vi "RT-TrapTest.vi"() -> ()   [LabVIEW 2010]
uses:
  <vilib>/userDefined/High Color/nirio_resource_hc.ctl
  <vilib>/rvi/interface/nirviOpenFPGA/nirviOpenFPGA.xnode
  C:/Users/HAGAR-IV/Desktop/HAGAR-V_Steuerung/Users/HAGAR-IV/Desktop/Johnny/pertrasgc fpga/FPGA-Trap-Test.vi
  <vilib>/rvi/ClientSDK/nirviWhatTheDeviceIsDoing.ctl
  <vilib>/rvi/interface/nirviReadWriteControl/nirviReadWriteControl.xnode
  <vilib>/rvi/interface/common/niFpgaNodeNameForErrorReporting.ctl
  <vilib>/rvi/errors/niLvFpgaWhatHappensToTopLevelVI.ctl
  <vilib>/rvi/interface/nirviMethod/nirviMethod.xnode
  <vilib>/rvi/interface/nirviCloseFPGA/nirviCloseFPGA.xnode
  <vilib>/FPGAPlugInAG/cRIO-9114/niLvFpga_Open_cRIO-9114.vi
  <vilib>/rvi/interface/common/dynamic/niFpgaDynamicAddResources.vi
  <vilib>/Utility/error.llb/Error Cluster From Error Code.vi
  <vilib>/rvi/errors/niLvFpgaAdjustHostInterfaceError.vi
  <vilib>/FPGAPlugInAG/Dynamic/niLvFpga_Close_Dynamic.vi
  NiFpgaLv.dll
panel:
  out "XY Graph":cluster{dbl[], dbl[]}(graph)
  out "Widrschtond":dbl
  in  "WerteMitteln":i32
  out "TempTrap":dbl
  in  "T(R)Koeff0":dbl=-251.0
  in  "T(R)Koeff2":dbl=-0.96
  in  "T(R)Koeff1":dbl=46.0
  out "WiderstandHeizdraht":dbl
  in  "Spannung":dbl=4.3
  in  "Präzisionswidrschtond":dbl=8.43
  in  "stop":bool
  in  "5VTrap1":bool
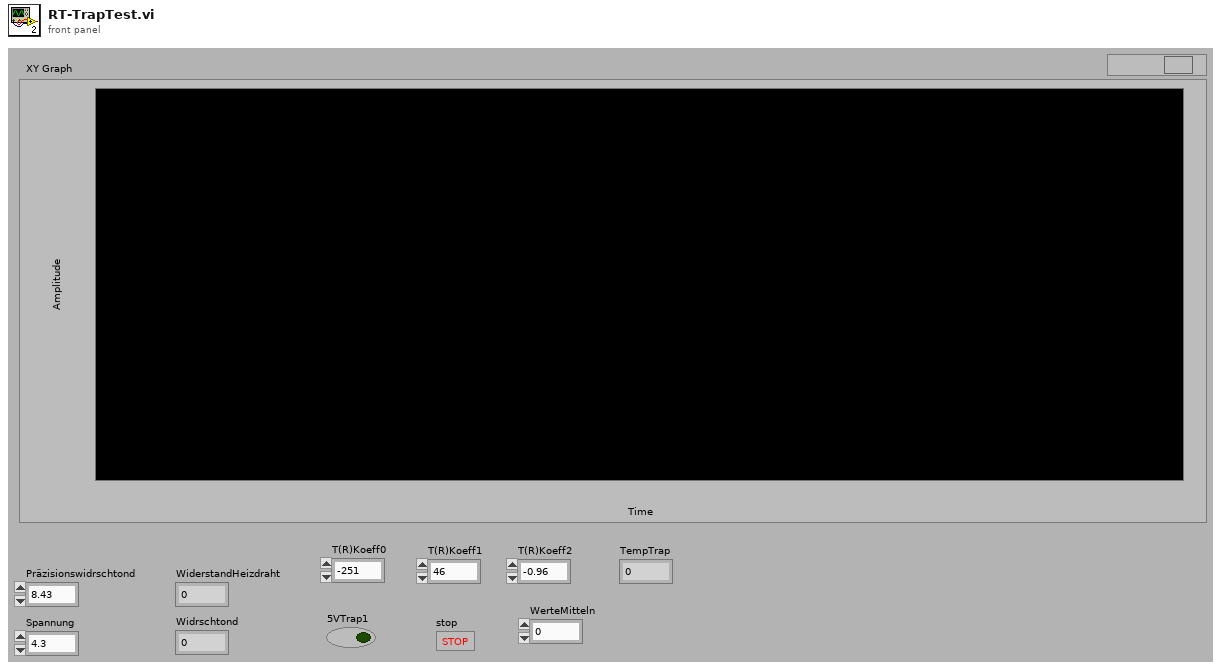
[diagram p1: front panel]
types:
  T1 = typedef "niFpgaNodeNameForErrorReporting.ctl" = enum16{"Open FPGA VI Reference", "Read/Write Control", "Invoke Method: Abort", "Invoke Method: Acknowledge IRQ", "Invoke Method: Download", "Invoke Method: FIFO.Configure", "Invoke Method: FIFO.Read", "Invoke Method: FIFO.Start", "Invoke Method: FIFO.Stop", "Invoke Method: FIFO.Write", "Invoke Method: Reset", "Invoke Method: Run", "Invoke Method: Wait on IRQ", "Close FPGA VI Reference"}
  T2 = typedef "niLvFpgaWhatHappensToTopLevelVI.ctl" = enum16{"top level VI scripted behind XNode", "top level VI inlined behind XNode"}
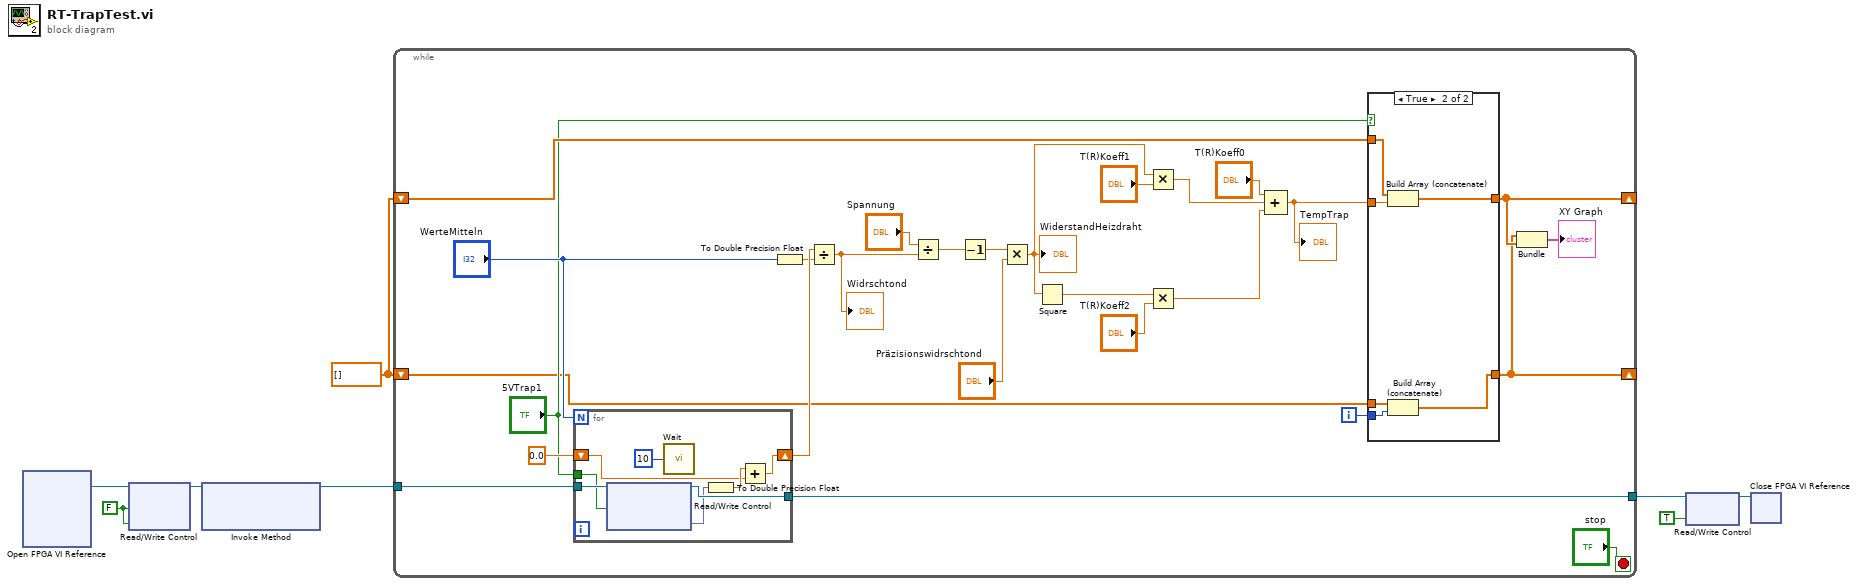
[diagram p0: block diagram]
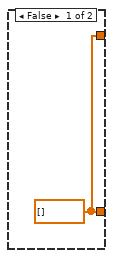
[diagram p2: hidden frame]
diagram:
  w1 = dbl[] []
  w7 = FALSE ("5VTrap1")
  n1 = xnode "Open FPGA VI Reference"() -> ("FPGA VI Reference Out"=w8:refnum<k20>)  [unwired: 2 in, 1 out]
  n2 = xnode "Read/Write Control"("FPGA VI Reference In"=w8, "5VTrap1"=w7, "stop"=w7) -> ("FPGA VI Reference Out"=w6:refnum<k20>)  [unwired: 1 in, 1 out]
  n3 = xnode "Invoke Method"("FPGA VI Reference In"=w6) -> ("FPGA VI Reference Out"=w5:refnum<k20>)  [unwired: 2 in, 1 out]
  n4 = while {
    tunnel: w5 -> [w35]
    tunnel: [w33] -> w4
    shift-right: [w13] -> _
    shift-left: w1 -> [w15]
    shift-right: [w9] -> _
    shift-left: w1 -> [w12]
    i -> [w11]
    stop <- "stop" stop-if-true
    n5 = for {
      N: "WerteMitteln" -> [_]
      tunnel: w35 -> [w50]
      tunnel: [w49] -> w33
      shift-right: [w45] -> w19
      shift-left: 0.0 -> [w46]
      tunnel: "5VTrap1" -> [w43]
      n6 = xnode "Read/Write Control"("FPGA VI Reference In"=w50, "5VTrap1"=w43) -> ("FPGA VI Reference Out"=w49:refnum<k20>, "AIWidrTrap1"=w48:fxp<+/-,26,5>)  [unwired: 1 in, 1 out]
      n7 = call "Wait"("Count(mSec)"=u32 10) -> ()  [unwired: 1 out]
      n8 = To Double Precision Float(number=w48) -> (double precision float=w47:dbl)
      n9 = Add(x=w47, y=w46) -> (x+y=w45:dbl)
    }
    n10 = To Double Precision Float(number="WerteMitteln") -> (double precision float=w18:dbl)
    n11 = Divide(x=w19, y=w18) -> (x/y=w17:dbl)
    "Widrschtond" <- w17
    n12 = Divide(x="Spannung", y=w17) -> (x/y=w31:dbl)
    n13 = Decrement(x=w31) -> (x-1=w30:dbl)
    n14 = Multiply(x=w30, y="Präzisionswidrschtond") -> (x*y=w27:dbl)
    "WiderstandHeizdraht" <- w27
    n15 = Square(x=w27) -> (x^2=w26:dbl)
    n16 = Multiply(x=w27, y="T(R)Koeff1") -> (x*y=w23:dbl)
    n17 = Multiply(x=w26, y="T(R)Koeff2") -> (x*y=w24:dbl)
    n18 = Compound Arithmetic op=ADD("T(R)Koeff0", w23, w24) -> (w16:dbl)
    "TempTrap" <- w16
    n19 = case shown="True" "5VTrap1" {
      tunnel: w16 -> [_ w39]
      tunnel: [w36 w42] -> w13
      tunnel: w15 -> [_ w40]
      tunnel: w12 -> [_ w41]
      tunnel: w11 -> [_ w38]
      tunnel: [w36 w37] -> w9
      frame False {
        w36 = dbl[] []
      }
      frame True {
        n20 = Build Array (concatenate)(w40, w39) -> (w42:dbl[])
        n21 = Build Array (concatenate)(w41, w38) -> (w37:dbl[])
      }
    }
    n22 = Bundle(w9, w13) -> (→"XY Graph":cluster{dbl[], dbl[]})  [unwired: 1 in]
  }
  n23 = xnode "Read/Write Control"("FPGA VI Reference In"=w4, "stop"=TRUE) -> ("FPGA VI Reference Out"=w2:refnum<k20>)  [unwired: 1 in, 1 out]
  n24 = xnode "Close FPGA VI Reference"("FPGA VI Reference In"=w2) -> ()  [unwired: 1 in, 1 out]
